vi "Add_Time_Seq.vi"(8 "Process Array":cluster{"Timing 0":dbl[]}[](array[cluster]), 11 "Initial State Array":cluster{"Timing 0":dbl[]}[](array[cluster])) -> (3 "Total Array":cluster{"Timing 0":dbl[]}[](array[cluster]))   [LabVIEW 2021]
panel:
  out "output array":dbl[](array[numeric])
  out "Timing 1":dbl[](array[numeric])
  out "Timing 0":dbl[](array[numeric])
  out "Port 2/line 6":cluster{"Timing 0":dbl[]}
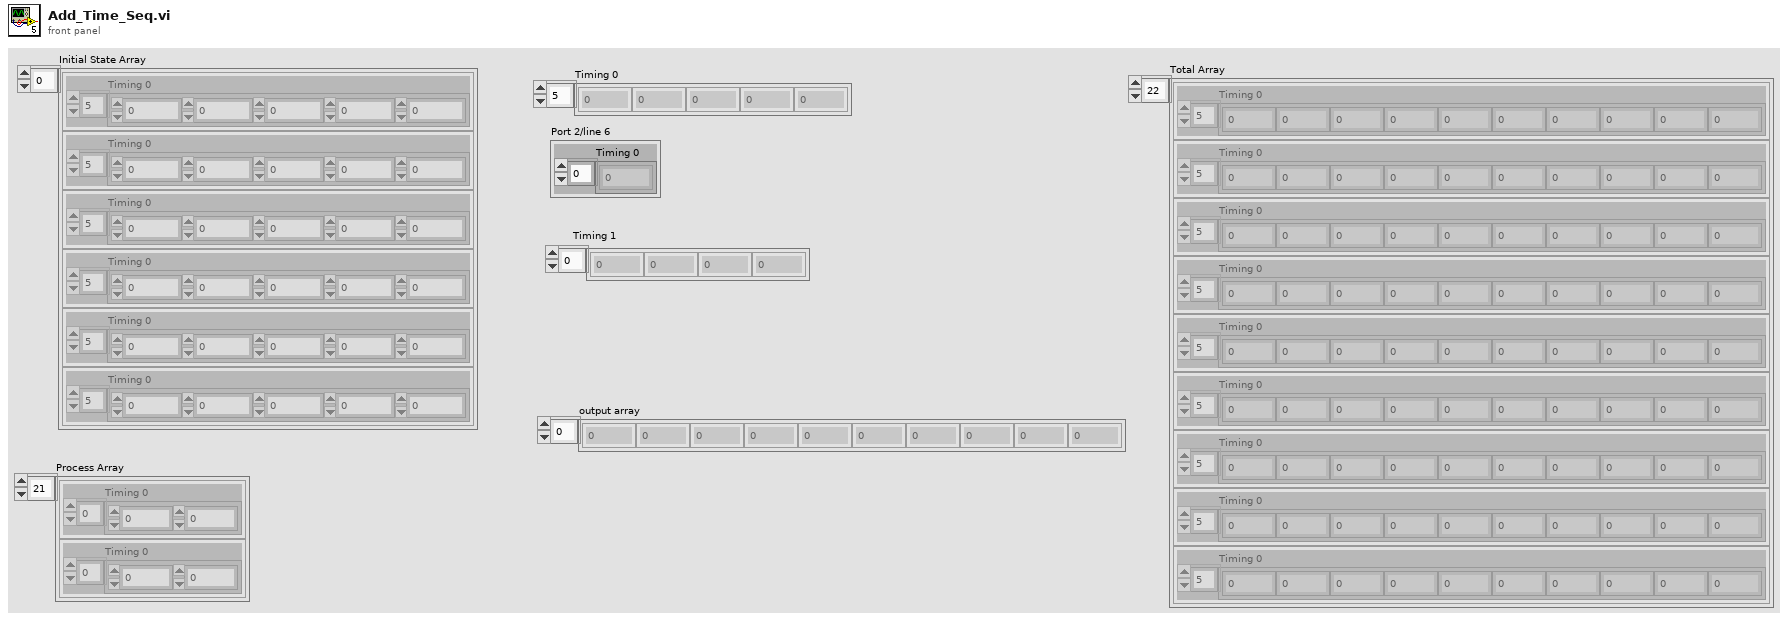
[diagram p1: front panel]
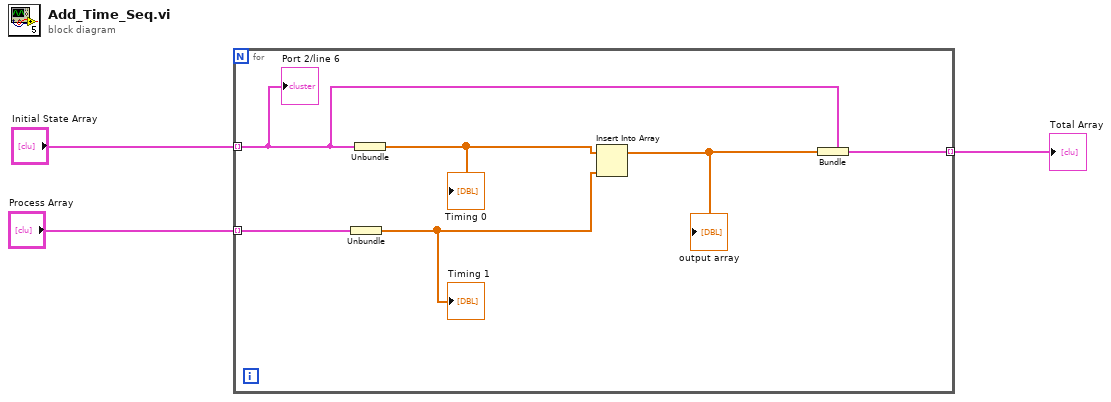
[diagram p0: block diagram]
diagram:
  n1 = for {
    tunnel: "Initial State Array" -> [w6] mode=indexing
    tunnel: "Process Array" -> [w9] mode=indexing
    tunnel: [w4] -> w1 mode=indexing
    n2 = Unbundle(w9) -> ("Timing 0"=w7:dbl[])
    "Timing 1" <- w7
    n3 = Unbundle(w6) -> ("Timing 0"=w8:dbl[])
    "Timing 0" <- w8
    n4 = Insert Into Array(array=w8, new element=w7) -> (w5:dbl[])  [unwired: 1 in]
    "output array" <- w5
    n5 = Bundle(cluster=w6, "Timing 0"=w5) -> (w4:cluster{"Timing 0":dbl[]})
    "Port 2/line 6" <- w6
  }
  "Total Array" <- w1
